vi "Add Node.vi"(8 "error in (no error)":errorcluster, 9 "Test Events":T1[](array[typedef]), 10 "Test Node":T2, 11 "Test Result in":refnum<class "Test Result.lvclass">) -> (0 "error out":errorcluster, 3 "Test Result out":refnum<class "Test Result.lvclass">)   [LabVIEW 2013, in "Caraya.lvlib" / "Test Result.lvclass"]
uses:
  Test Result.lvclass
  Test Node.ctl
  Test Registration Data.ctl
  Assert Event Data.ctl
  Test Result.lvclass/Test Result.ctl
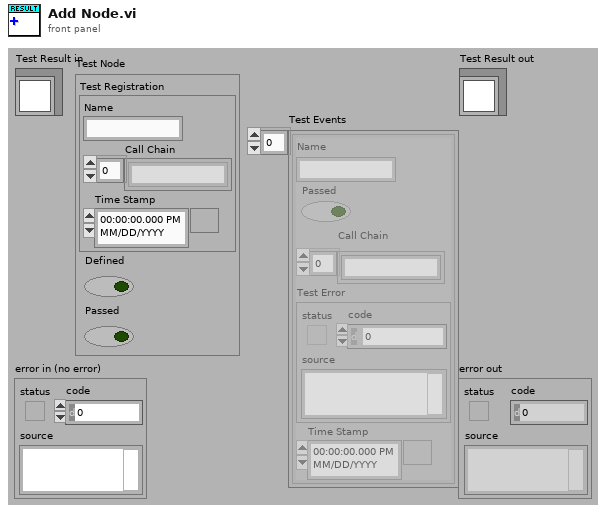
[diagram p1: front panel]
types:
  T1 = typedef "Caraya.lvlib/Test Result.lvclass/Assert Event Data.ctl" = cluster{"Name":string, "Passed":bool, "Call Chain":string[], "Test Error":errorcluster, "Time Stamp":timestamp}
  T2 = typedef "Caraya.lvlib/Test Result.lvclass/Test Node.ctl" = cluster{"Test Registration":T3, "Defined":bool, "Passed":bool}
  T3 = typedef "Caraya.lvlib/Test Result.lvclass/Test Registration Data.ctl" = cluster{"Name":string, "Call Chain":string[], "Time Stamp":timestamp}
  T4 = typedef "Caraya.lvlib/Test Result.lvclass/Node Results.ctl" = cluster{"Node":T2, "Assertions":T1[]}
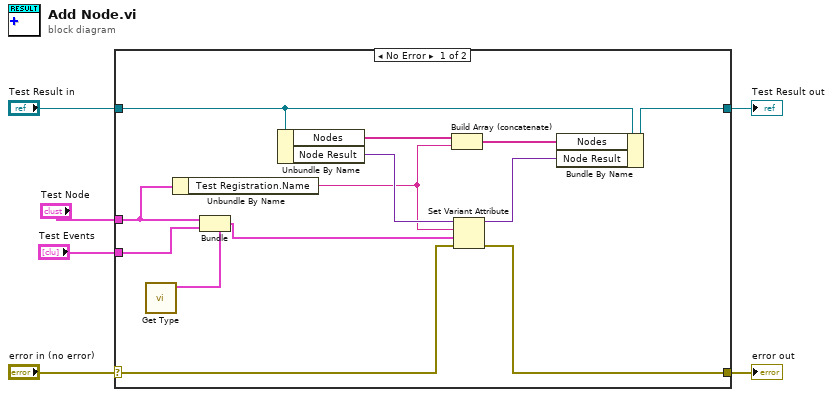
[diagram p0: block diagram]
diagram:
  n1 = case shown="No Error" "error in (no error)" {
    selector: "error in (no error)" -> [w8 w21]
    tunnel: [w7 w21] -> w5
    tunnel: [w17 w20] -> w3
    tunnel: "Test Result in" -> [w18 w20]
    tunnel: "Test Node" -> [w13 _]
    tunnel: "Test Events" -> [w19 _]
    frame No Error {
      n2 = call "Get Type.vi"() -> ("Node Result"=w16:T4)  [unwired: 11 in]
      n3 = Unbundle By Name(w13) -> ("Test Registration.Name"=w11:string)
      n4 = Bundle(cluster=w16, "Node"=w13, "Assertions"=w19) -> (w10:T4)
      n5 = Unbundle By Name(w18) -> ("Nodes"=w15:string[], "Node Result"=w12:variant)
      n6 = Build Array (concatenate)(w15, w11) -> (w14:string[])
      n7 = Set Variant Attribute(Variant=w12, name=w11, value=w10, error in=w8) -> (Variant out=w9:variant, error out=w7:errorcluster)  [unwired: 1 out]
      n8 = Bundle By Name(cluster=w18, "Nodes"=w14, "Node Result"=w9) -> (w17:refnum<class "Test Result.lvclass">)
    }
    frame Error {
    }
  }
  "error out" <- w5
  "Test Result out" <- w3
